vi "configuration UI.vi"() -> ()   [LabVIEW 2015, in "Scaling editor node.lvclass"]
uses:
  Scaling editor node.lvclass
  <vilib>/NI/Configuration Framework/Node/NodeRef.ctl
  <vilib>/NI/Configuration Framework/Node/NISE_CEF_Node.lvclass
  <vilib>/NI/AMC/Message Queue.ctl
  <vilib>/NI/AMC/Message.ctl
  <vilib>/NI/Tools/Keyed Array/KeyedArray.ctl
  <vilib>/NI/Configuration Framework/Node/UserEventRef.ctl
  <vilib>/NI/Configuration Framework/Controls/EventCluster.ctl
  <vilib>/NI/Configuration Framework/Node/StopEvent.ctl
  <vilib>/NI/Configuration Framework/Node/RefreshUIEvent.ctl
  <vilib>/NI/Configuration Framework/Node/CacheState.ctl
  <vilib>/NI/Configuration Framework/Node/NodeChangeEvent.ctl
  module/configuration/controls/scale data types.ctl
  <vilib>/NI/DCAF UI Toolkit/Controls/Add.ctl
  <vilib>/NI/DCAF UI Toolkit/Controls/Remove.ctl
  <vilib>/NI/DCAF Table API/Table Manager/references.ctl
  <vilib>/NI/DCAF/Tag Editor Core/control module/editor node/channel action event.ctl
  <vilib>/NI/DCAF/Tag Editor Core/control module/editor node/dialog output action.ctl
  <vilib>/NI/Tag Bus Module Framework/channel/TBM channel.lvclass
  <vilib>/NI/Tag Bus/tag/tag descriptor.lvclass
  <vilib>/Utility/miscctls.llb/LVPositionTypeDef.ctl
  <vilib>/NI/DCAF Table API/Listbox/Multi Column Listbox.lvclass
  <vilib>/NI/DCAF/Tag Editor Core/control module/editor node/control module editor.lvclass
  <vilib>/NI/Tools/Keyed Array/Tools_KeyedArray.lvlib
  <vilib>/NI/AMC/AMC.lvlib
  <vilib>/NI/Configuration Framework/NISE_CEF_TreeControl.lvlib
  <vilib>/NI/DCAF Table API/Table Manager/Table Manager.lvclass
  <vilib>/NI/DCAF UI Toolkit/Controls/DCAF UI Elements.lvlib
  module/configuration/Scaling configuration.lvclass
panel:
  in  "scale data types":T1
  in  "Top Level Tab Control":enum32{"Scaling Module"}(tab)
  in  "Sub Tab Control":enum32{"Mappings", "Scale Configuration"}(tab)
  in  "Remove Mapping":T2
  in  "Add Mapping":T3
  in  "Multicolumn Listbox":i32(listbox)
  in  "Scales":i32(listbox)
  in  "Add Scale":T3
  in  "Remove Scale":T2
  in  "node change":T4
  in  "cache state":T5
  in  "refresh UI":T6
  in  "stop event":T7
  in  "user event":T8
  in  "main queue":T9
  in  "node ref":T10
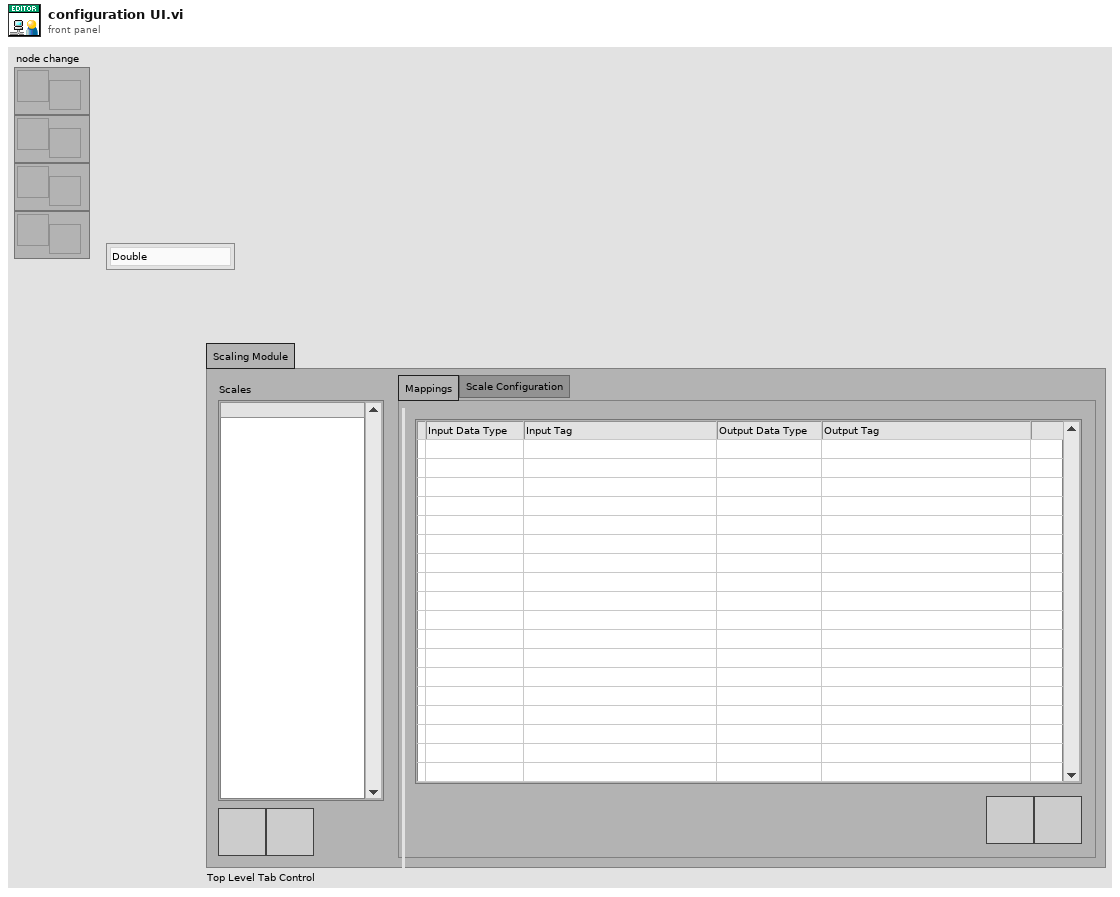
[diagram p1: front panel]
types:
  T1 = typedef "Scaling configuration.lvclass/scale data types.ctl" = enum16{"Double", "Single", "I64", "I32", "I16", "I8", "U64", "U32", "U16", "U8"}
  T2 = typedef "DCAF UI Elements.lvlib/Remove.ctl" = bool
  T3 = typedef "DCAF UI Elements.lvlib/Add.ctl" = bool
  T4 = typedef "NISE_CEF_Node.lvclass/NodeChangeEvent.ctl" = refnum<user-event>
  T5 = typedef "NISE_CEF_Node.lvclass/CacheState.ctl" = refnum<user-event>
  T6 = typedef "NISE_CEF_Node.lvclass/RefreshUIEvent.ctl" = refnum<user-event>
  T7 = typedef "NISE_CEF_Node.lvclass/StopEvent.ctl" = refnum<user-event>
  T8 = typedef "NISE_CEF_Node.lvclass/UserEventRef.ctl" = refnum<user-event>
  T9 = typedef "AMC.lvlib/Message Queue.ctl" = refnum<queue>
  T10 = typedef "NISE_CEF_Node.lvclass/NodeRef.ctl" = refnum<data-value>
  T11 = typedef "LVPositionTypeDef.ctl" = cluster{"Left":i32, "Top":i32}
  T12 = typedef "Table Manager.lvlib/Table Manager.lvclass/references.ctl" = cluster{"stop event":T7, "refresh UI":T6, "cache state":T5, "node change":T4, "user event out":refnum<user-event>, "main queue":T9, "user event":T8}
  T13 = typedef "Table Manager.lvlib/Table Manager.lvclass/object ref.ctl" = cluster{"engine":refnum<data-value>, "Node Ref":refnum<data-value>}
  T14 = typedef "LVRowAndColumnTypeDef.ctl" = cluster{"Row":i32, "Column":i32}
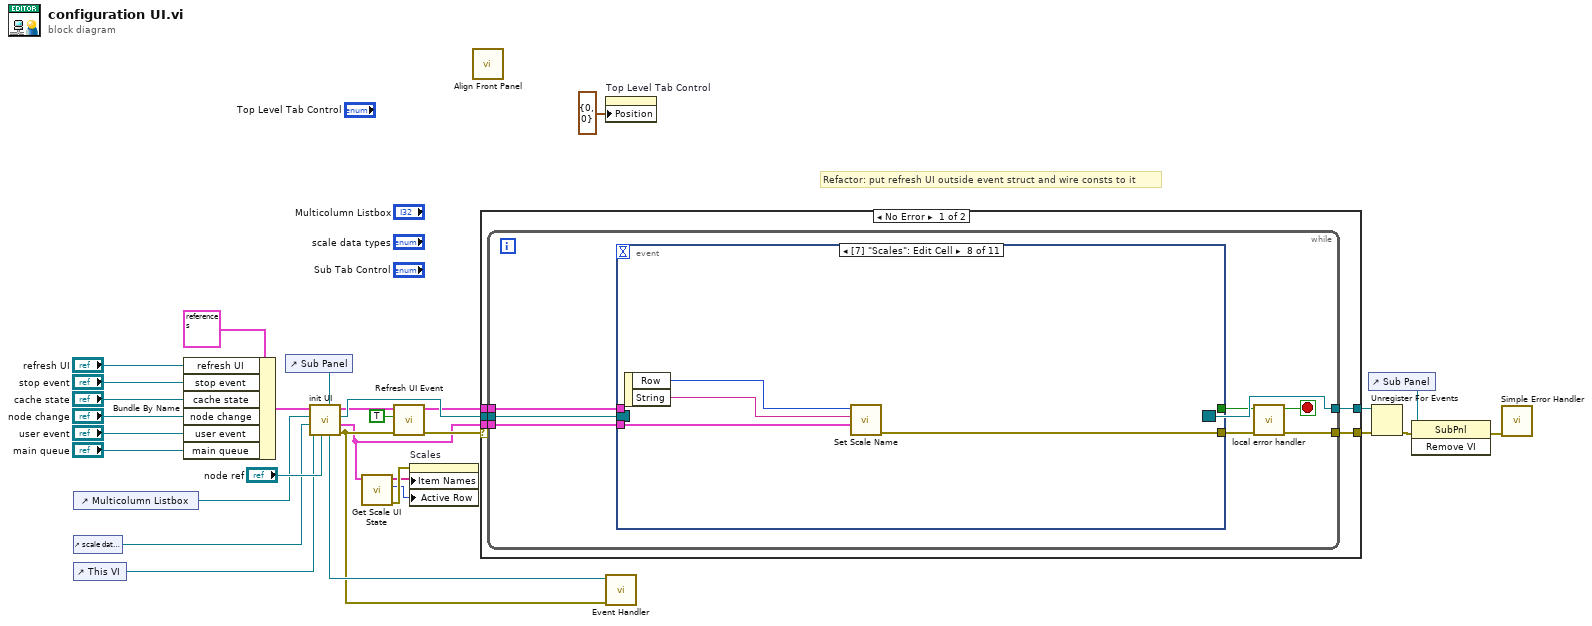
[diagram p0: block diagram]
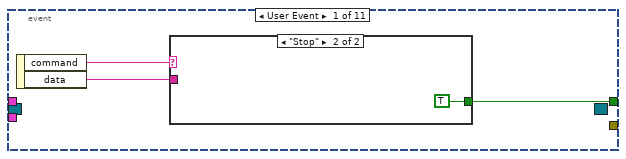
[diagram p2: hidden frame]
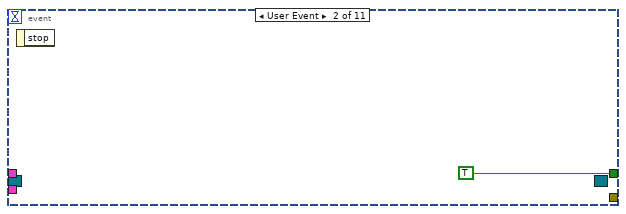
[diagram p4: hidden frame]
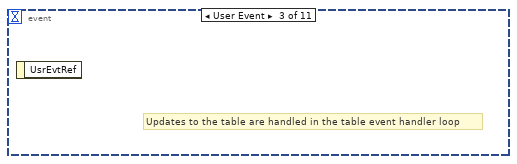
[diagram p5: hidden frame]
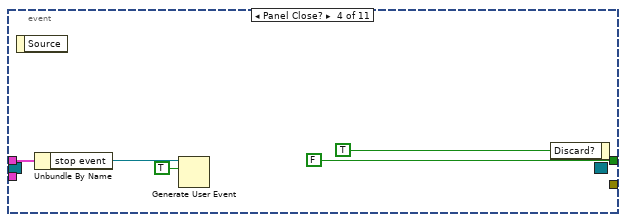
[diagram p6: hidden frame]
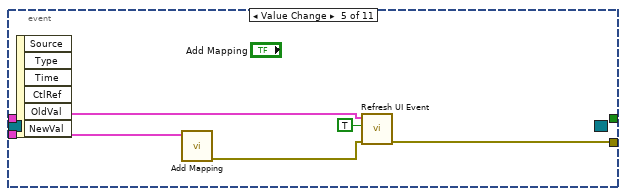
[diagram p7: hidden frame]
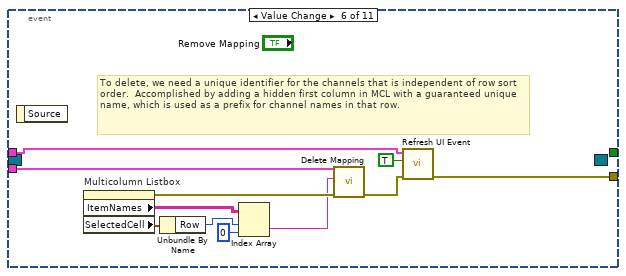
[diagram p8: hidden frame]
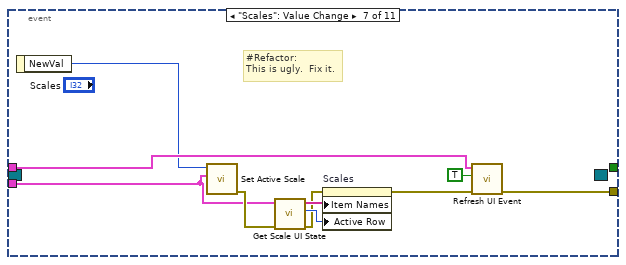
[diagram p9: hidden frame]
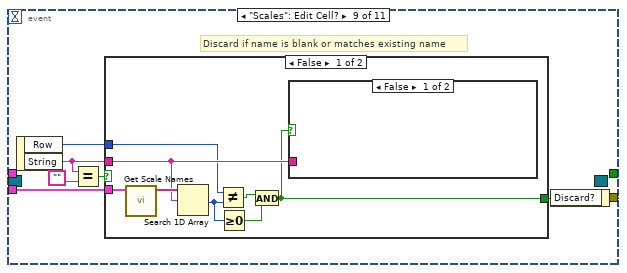
[diagram p10: hidden frame]
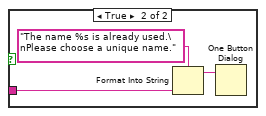
[diagram p11: hidden frame]
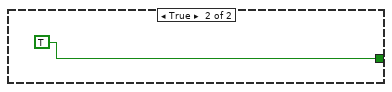
[diagram p12: hidden frame]
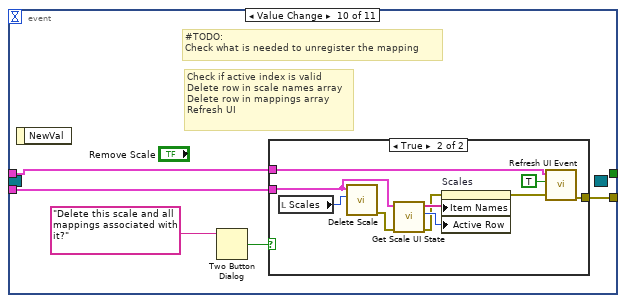
[diagram p13: hidden frame]
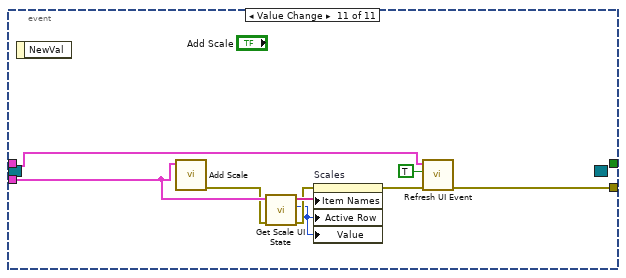
[diagram p15: hidden frame]
diagram:
  # "Refactor: put refresh UI outside event struct and wire consts to it"
  n1 = control-ref of="Multicolumn Listbox"() -> (w6:refnum<vi>)
  n2 = control-ref of="scale data types"() -> (w8:refnum<vi>)
  n3 = control-ref of="This VI"() -> (w7:refnum<vi>)
  n4 = Bundle By Name(cluster=T12 {"stop event"=refnum, "refresh UI"=refnum, "cache state"=refnum, "node change"=refnum, "user event out"=refnum, "main queue"=refnum, "user event"=refnum} ("References in"), "refresh UI"="refresh UI", "stop event"="stop event", "cache state"="cache state", "node change"="node change", "user event"="user event", "main queue"="main queue") -> (w15:T12)
  n5 = control-ref of="Sub Panel"() -> (w11:refnum<vi>)
  n6 = call "init UI.vi"("Sub Panel"=w11, "node ref"="node ref", "Top VI"=w7, "Enum in"=w8, "Listbox"=w6, "References in"=w15) -> ("error out"=w9:errorcluster, "Objects out"=w2:T13, "Event Registration Refnum"=w20:refnum<event-registration>, "References out"=w17:T12, "Multi Column Listbox out"=w10:refnum<class "Multi Column Listbox.lvclass">)  [unwired: 1 in]
  n7 = call "Get Scale UI State.vi"("references"=w2) -> ("error out"=w5:errorcluster, "active scale index"=w4:i32, "scale names"=w3:string[])  [unwired: 8 in]
  n8 = call "Refresh UI Event.vi"("error in"=w9, "Refresh?"=TRUE, "References in"=w17) -> ("error out"=w19:errorcluster, "References out"=w16:T12)  [unwired: 7 in]
  n9 = property on="Scales" class="LstBox (strict)"(error in=w5, "Item Names"=w3, "Active Row"=w4) -> ()  [unwired: 1 in, 2 out]
  n10 = call <vilib>:"Align Front Panel.vi"() -> ()  [unwired: 10 in, 2 out]
  n11 = case shown="No Error" w19 {
    selector: w19 -> [_ w127]
    tunnel: w20 -> [w35 w126]
    tunnel: [w34 w126] -> w30
    tunnel: [w33 w127] -> w29
    tunnel: w2 -> [w31 _]
    tunnel: w16 -> [w32 _]
    frame No Error {
      n12 = while {
        tunnel: w35 -> [w43]
        tunnel: [w42] -> w34
        tunnel: [w39] -> w33
        tunnel: w32 -> [w38]
        tunnel: w31 -> [w37]
        stop <- w41 stop-if-true
        n13 = event shown="[7] \"Scales\": Edit Cell" {
          selector: w43 -> [_ _ _ _ _ _ _ _ _ _ _]
          dyn-events: [_ _ _ _ _ _ _ _ _ _ _] -> w42
          timeout: _ -> [_ _ _ _ _ _ _ _ _ _ _]
          tunnel: [w46 TRUE _ FALSE _ _ _ _ _ _ _] -> w40
          tunnel: w38 -> [_ _ _ w50 w56 w67 w78 _ _ w105 w124]
          tunnel: w37 -> [_ _ _ _ w55 w66 w71 w81 w87 w102 w119]
          tunnel: [_ _ _ _ w58 w69 w79 w80 _ w106 w123] -> w36
          event User Event {
            n14 = event-data() -> ("command"=w45:string, "data"=w44:string)  [unwired: 1 in]
            n15 = case shown="\"Stop\"" w45 {
              tunnel: [_ TRUE] -> w46
              tunnel: w44 -> [_ _]
              frame Default {
              }
              frame "Stop" {
              }
            }
          }
          event User Event {
            n16 = event-data() -> ()  [unwired: 1 in, 1 out]
          }
          event User Event {
            # "Updates to the table are handled in the table event handler loop"
            n17 = event-data() -> ()  [unwired: 1 in, 1 out]
          }
          event Panel Close? {
            n18 = event-data() -> ()  [unwired: 1 in, 1 out]
            n19 = Unbundle By Name(w50) -> ("stop event"=w49:T7)
            n20 = Generate User Event(user event=w49, event data cluster=TRUE ("event data")) -> ()  [unwired: 2 in, 2 out]
            n21 = event-data("Discard?"=TRUE) -> ()  [unwired: 1 in, 1 out]
          }
          event Value Change {
            n22 = event-data() -> ()  [unwired: 1 in, 6 out]
            n23 = call "Add Mapping.vi"("references"=w55) -> ("error out"=w54:errorcluster)  [unwired: 9 in, 1 out]
            n24 = call "Refresh UI Event.vi"("error in"=w54, "Refresh?"=TRUE, "References in"=w56) -> ("error out"=w58:errorcluster)  [unwired: 7 in, 1 out]
          }
          event Value Change {
            # "To delete, we need a unique identifier for the channels that is independent of row sort order.  Accomplished by adding a hidden first column in MCL with a guaranteed unique name, which is used as a prefix for channel names in that row."
            n25 = event-data() -> ()  [unwired: 1 in, 1 out]
            n26 = property on="Multicolumn Listbox" class="MCListbox (strict)"() -> (error out=w64:errorcluster, "ItemNames"=w62:string[][], "SelectedCell"=w63:T14)  [unwired: 2 in, 1 out]
            n27 = Unbundle By Name(w63) -> ("Row"=w60:i32)
            n28 = Index Array(array=w62, index (row)=w60, index (col)=0 ("disabled index (col)")) -> (element=w59:string)
            n29 = call "Delete Mapping.vi"("error in (no error)"=w64, "Row Name"=w59, "references"=w66) -> ("error out"=w65:errorcluster)  [unwired: 7 in, 1 out]
            n30 = call "Refresh UI Event.vi"("error in"=w65, "Refresh?"=TRUE, "References in"=w67) -> ("error out"=w69:errorcluster)  [unwired: 7 in, 1 out]
          }
          event "Scales": Value Change {
            # "#Refactor:\nThis is ugly.  Fix it."
            n31 = event-data() -> ("NewVal"=w77:i32)  [unwired: 1 in]
            n32 = call "Set Active Scale.vi"("references"=w71, "Index"=w77) -> ("error out"=w72:errorcluster)  [unwired: 9 in]
            n33 = call "Get Scale UI State.vi"("error in (no error)"=w72, "references"=w71) -> ("error out"=w73:errorcluster, "active scale index"=w74:i32, "scale names"=w75:string[])  [unwired: 7 in]
            n34 = property on="Scales" class="LstBox (strict)"(error in=w73, "Item Names"=w75, "Active Row"=w74) -> (error out=w70:errorcluster)  [unwired: 1 in, 1 out]
            n35 = call "Refresh UI Event.vi"("error in"=w70, "Refresh?"=TRUE, "References in"=w78) -> ("error out"=w79:errorcluster)  [unwired: 7 in, 1 out]
          }
          event "Scales": Edit Cell {
            n36 = event-data() -> ("Row"=w83:i32, "String"=w82:string)  [unwired: 1 in]
            n37 = call "Set Scale Name.vi"("references"=w81, "name"=w82, "index"=w83) -> ("error out"=w80:errorcluster)  [unwired: 8 in]
          }
          event "Scales": Edit Cell? {
            # "Discard if name is blank or matches existing name"
            n38 = event-data() -> ("Row"=w84:i32, "String"=w86:string)  [unwired: 1 in]
            n39 = Equal?(x=w86, y="") -> (x = y?=w89:bool)
            n40 = case shown="False" w89 {
              tunnel: [w90 TRUE] -> w88
              tunnel: w87 -> [w97 _]
              tunnel: w86 -> [w95 _]
              tunnel: w84 -> [w94 _]
              frame False {
                n41 = call "Get Scale Names.vi"("references"=w97) -> ("scale names"=w96:string[])  [unwired: 9 in, 1 out]
                n42 = Search 1D Array(1D array=w96, element=w95) -> (index of element=w93:i32)  [unwired: 1 in]
                n43 = Not Equal?(x=w94, y=w93) -> (x != y?=w92:bool)
                n44 = Greater Or Equal To 0?(x=w93) -> (x >= 0?=w91:bool)
                n45 = And(x=w92, y=w91) -> (x .and. y?=w90:bool)
                n46 = case shown="False" w90 {
                  tunnel: w95 -> [_ w98]
                  frame False {
                  }
                  frame True {
                    n47 = Format Into String(format string="The name %s is already used.\nPlease choose a unique name.", w98) -> (resulting string=w100:string)  [unwired: 2 in, 1 out]
                    n48 = One Button Dialog(message=w100) -> ()  [unwired: 1 in, 1 out]
                  }
                }
              }
              frame True {
              }
            }
            n49 = event-data("Discard?"=w88) -> ()  [unwired: 1 in, 1 out]
          }
          event Value Change {
            # "#TODO:\nCheck what is needed to unregister the mapping"
            # "Check if active index is valid\nDelete row in scale names array\nDelete row in mappings array\nRefresh UI"
            n50 = event-data() -> ()  [unwired: 1 in, 1 out]
            n51 = Two Button Dialog(message="Delete this scale and all mappings associated with it?" ("format string")) -> (T button?=w103:bool)  [unwired: 2 in]
            n52 = case shown="True" w103 {
              tunnel: [_ w116] -> w106
              tunnel: w105 -> [_ w114]
              tunnel: w102 -> [_ w109]
              frame False {
              }
              frame True {
                n53 = local read "Scales"() -> (w113:i32)
                n54 = call "Delete Scale.vi"("Index"=w113, "references"=w109) -> ("error out"=w108:errorcluster)  [unwired: 9 in]
                n55 = call "Get Scale UI State.vi"("error in (no error)"=w108, "references"=w109) -> ("error out"=w110:errorcluster, "active scale index"=w111:i32, "scale names"=w112:string[])  [unwired: 7 in]
                n56 = property on="Scales" class="LstBox (strict)"(error in=w110, "Item Names"=w112, "Active Row"=w111) -> (error out=w107:errorcluster)  [unwired: 1 in, 1 out]
                n57 = call "Refresh UI Event.vi"("error in"=w107, "Refresh?"=TRUE, "References in"=w114) -> ("error out"=w116:errorcluster)  [unwired: 7 in, 1 out]
              }
            }
          }
          event Value Change {
            n58 = event-data() -> ()  [unwired: 1 in, 1 out]
            n59 = call "Add Scale.vi"("references"=w119) -> ("error out"=w118:errorcluster)  [unwired: 10 in]
            n60 = call "Get Scale UI State.vi"("error in (no error)"=w118, "references"=w119) -> ("error out"=w121:errorcluster, "active scale index"=w117:i32, "scale names"=w122:string[])  [unwired: 7 in]
            n61 = property on="Scales" class="LstBox (strict)"(error in=w121, "Item Names"=w122, "Active Row"=w117, "Value"=w117) -> (error out=w120:errorcluster)  [unwired: 1 in, 1 out]
            n62 = call "Refresh UI Event.vi"("error in"=w120, "Refresh?"=TRUE, "References in"=w124) -> ("error out"=w123:errorcluster)  [unwired: 7 in, 1 out]
          }
        }
        n63 = call "local error handler.vi"("error in (no error)"=w36, "Boolean in"=w40) -> ("error out"=w39:errorcluster, "Boolean out"=w41:bool)  [unwired: 8 in]
      }
    }
    frame Error {
    }
  }
  n64 = property on="Top Level Tab Control" class="TabCtl (strict)"("Position"=T11 {"Left"=0, "Top"=0}) -> ()  [unwired: 2 in, 2 out]
  n65 = call-dynamic "Event Handler.vi"("error in"=w9, "Listbox in"=w10) -> ()  [unwired: 8 in, 2 out]
  n66 = control-ref of="Sub Panel"() -> (w14:refnum<vi>)
  n67 = Unregister For Events(event registration refnum=w30, error in=w29) -> (error out=w13:errorcluster)
  n68 = invoke class="SubPnl" method="Remove VI"(reference=w14, error in=w13) -> (error out=w12:errorcluster)  [unwired: 1 in, 2 out]
  n69 = call <vilib>:"Simple Error Handler.vi"("error in (no error)"=w12) -> ()  [unwired: 4 in, 5 out]
